vi "Jain's Interpolation Method.vi"(10 "FFT array":dbl[](array[numeric])) -> (0 "max index(es)":i32, 2 "Index Bin":dbl)   [LabVIEW 2014]
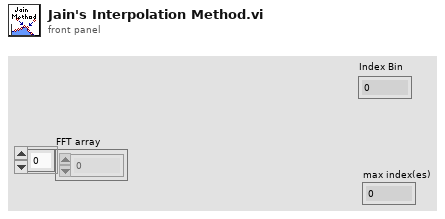
[diagram p1: front panel]
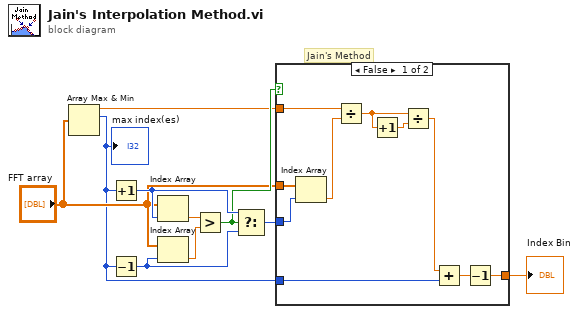
[diagram p0: block diagram]
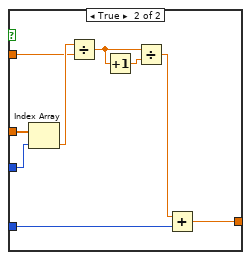
[diagram p2: hidden frame]
diagram:
  # "Jain's Method"
  n1 = Array Max & Min(array="FFT array") -> (max value=w3:dbl, max index (indices)=w2:i32)  [unwired: 2 out]
  "max index(es)" <- w2
  n2 = Increment(x=w2) -> (x+1=w7:i32)
  n3 = Decrement(x=w2) -> (x-1=w8:i32)
  n4 = Index Array(array="FFT array", index=w7) -> (element=w10:dbl)
  n5 = Index Array(array="FFT array", index=w8) -> (element=w9:dbl)
  n6 = Greater?(x=w10, y=w9) -> (0:w6:bool)
  n7 = Select(t=w7, s=w6, f=w8) -> (s? t:f=w5:i32)
  n8 = case shown="False" w6 {
    tunnel: w5 -> [w19 w28]
    tunnel: "FFT array" -> [w18 w29]
    tunnel: w3 -> [w20 w26]
    tunnel: w2 -> [w11 w22]
    tunnel: [w14 w21] -> w1
    frame False {
      n9 = Index Array(array=w18, index=w19) -> (element=w17:dbl)
      n10 = Divide(x=w20, y=w17) -> (x/y=w15:dbl)
      n11 = Increment(x=w15) -> (x+1=w16:dbl)
      n12 = Divide(x=w15, y=w16) -> (x/y=w12:dbl)
      n13 = Add(x=w12, y=w11) -> (x+y=w13:dbl)
      n14 = Decrement(x=w13) -> (x-1=w14:dbl)
    }
    frame True {
      n15 = Index Array(array=w29, index=w28) -> (element=w27:dbl)
      n16 = Divide(x=w27, y=w26) -> (x/y=w24:dbl)
      n17 = Increment(x=w24) -> (x+1=w25:dbl)
      n18 = Divide(x=w24, y=w25) -> (x/y=w23:dbl)
      n19 = Add(x=w23, y=w22) -> (x+y=w21:dbl)
    }
  }
  "Index Bin" <- w1
